vi "INST_PS_MEAS_3.0.0.vi"(0 "VISA session":refnum<visa-resource-name>="TCPIP0::169.254.70.130::inst0::INSTR", 1 "Clear Error in":bool, 3 "SEL_PS":string(combo)="PS1", 7 "Channel Name (1)":string="3", 11 "error in (no error)":errorcluster, 12 "Measurement Type (1: Voltage)":i32(ring)=1 items=["Current", "Voltage"], 14 "Use OPC?(T)":bool=TRUE) -> (4 "dup VISA session":refnum<visa-resource-name>="TCPIP0::169.254.70.130::inst0::INSTR", 6 "Measurement":dbl=28.01386 format="%.2p", 10 "Measurement (str)":string="+2.801386E+01\n", 15 "error out":errorcluster)   [LabVIEW 2018]
doc: "This VI takes a measurement on the output signal and returns the measured value."
uses:
  Initialize References/Station References Global.vi
panel:
  in  "General Settings:Timeout Value":u32=2000
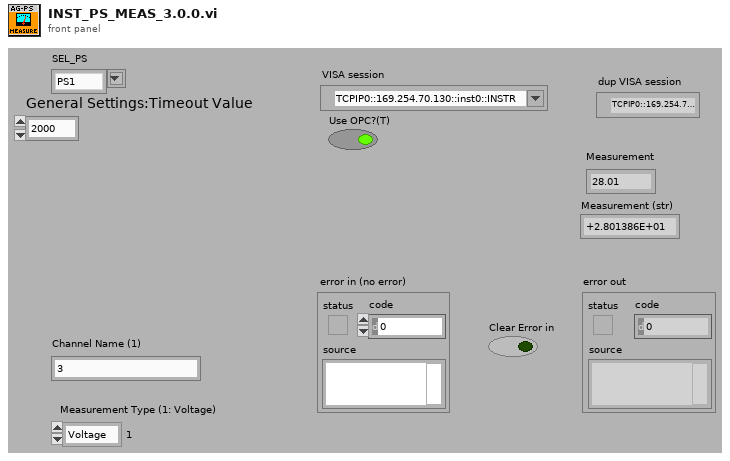
[diagram p1: front panel]
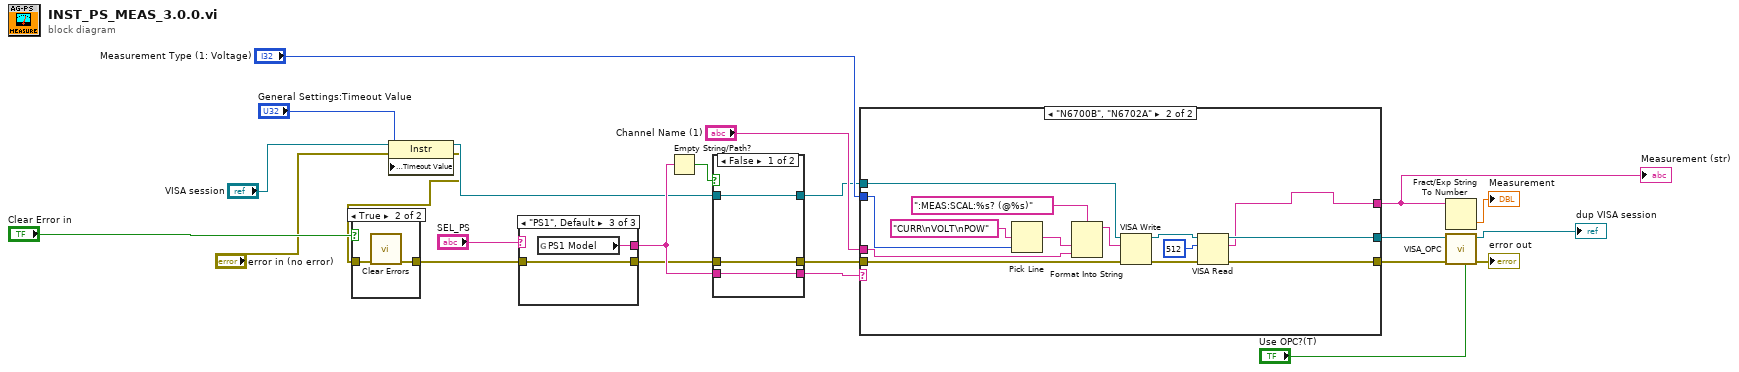
[diagram p0: block diagram]
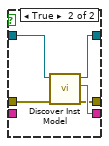
[diagram p2: hidden frame]
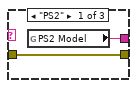
[diagram p3: hidden frame]
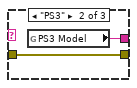
[diagram p4: hidden frame]
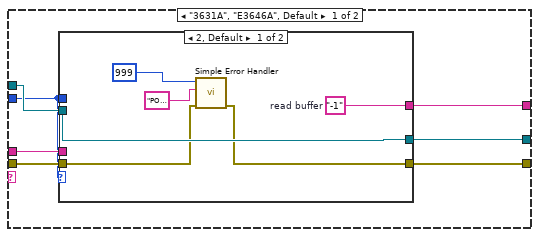
[diagram p5: hidden frame]
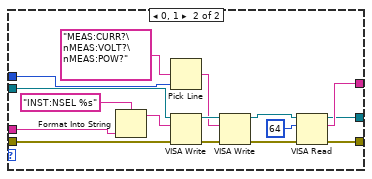
[diagram p6: hidden frame]
diagram:
  n1 = property class="Instr"(reference="VISA session", error in="error in (no error)", "General Settings:Timeout Value"="General Settings:Timeout Value") -> (reference out=w4:refnum<visa-resource-name>, error out=w3:errorcluster)
  n2 = case shown="True" "Clear Error in" {
    tunnel: w3 -> [w24 w26]
    tunnel: [w24 w25] -> w11
    frame False {
    }
    frame True {
      n3 = call <vilib>:"Clear Errors.vi"("error in (no error)"=w26) -> ("error out"=w25:errorcluster)  [unwired: 5 in, 1 out]
    }
  }
  n4 = case shown="\"PS1\", Default" "SEL_PS" {
    tunnel: [w28 w30 w32] -> w14
    tunnel: w11 -> [w27 w29 w31]
    tunnel: [w27 w29 w31] -> w13
    frame "PS2" {
      n5 = global read "Station References Global.vi" "PS2 Model"() -> (w28:string)
    }
    frame "PS3" {
      n6 = global read "Station References Global.vi" "PS3 Model"() -> (w30:string)
    }
    frame "PS1", Default {
      n7 = global read "Station References Global.vi" "PS1 Model"() -> (w32:string)
    }
  }
  n8 = Empty String/Path?(string/path=w14) -> (empty?=w15:bool)
  n9 = case shown="False" w15 {
    tunnel: [w35 w40] -> w9
    tunnel: w14 -> [w35 _]
    tunnel: [w34 w39] -> w10
    tunnel: w13 -> [w34 w38]
    tunnel: w4 -> [w33 w37]
    tunnel: [w33 w36] -> w8
    frame False {
    }
    frame True {
      n10 = call "Discover Inst Model.vi"("error in"=w38, "Session In"=w37) -> ("error out"=w39:errorcluster, "Model #"=w40:string, "Session Out"=w36:refnum<visa-resource-name>)  [unwired: 7 in]
    }
  }
  n11 = case shown="\"N6700B\", \"N6702A\"" w9 {
    tunnel: [w47 w71] -> w1
    tunnel: w8 -> [w46 w76]
    tunnel: [w45 w70] -> w23
    tunnel: [w44 w73] -> w20
    tunnel: w10 -> [w43 w72]
    tunnel: "Measurement Type (1: Voltage)" -> [w41 w75]
    tunnel: "Channel Name (1)" -> [w42 w74]
    frame "3631A", "E3646A", Default {
      n12 = case shown="2, Default" w41 {
        tunnel: [w52 w67] -> w47
        tunnel: w46 -> [w53 w61]
        tunnel: [w50 w60] -> w45
        tunnel: [w53 w59] -> w44
        tunnel: w43 -> [w51 w58]
        tunnel: w42 -> [_ w57]
        tunnel: w41 -> [_ w54]
        frame 2, Default {
          w52 = "-1"  # read buffer
          n13 = call <vilib>:"Simple Error Handler.vi"("error code (no error:0)"=999, "error source (\" \")"="POWER MEAS NOT AVAILABLE ON THIS MODEL OF PS" ("error source (\" \")"), "error in (no error)"=w51) -> ("error out"=w50:errorcluster)  [unwired: 2 in, 4 out]
        }
        frame 0, 1 {
          n14 = Format Into String(format string="INST:NSEL %s", w57) -> (resulting string=w64:string)  [unwired: 2 in, 1 out]
          n15 = Pick Line(multi-line string="MEAS:CURR?\nMEAS:VOLT?\nMEAS:POW?", line index=w54) -> (output string=w55:string)  [unwired: 1 in]
          n16 = VISA Write(VISA resource name=w61, write buffer=w64, error in (no error)=w58) -> (VISA resource name out=w62:refnum<visa-resource-name>, error out=w63:errorcluster)  [unwired: 1 out]
          n17 = VISA Write(VISA resource name=w62, write buffer=w55, error in (no error)=w63) -> (VISA resource name out=w66:refnum<visa-resource-name>, error out=w69:errorcluster)  [unwired: 1 out]
          n18 = VISA Read(VISA resource name=w66, byte count=u32 64, error in (no error)=w69) -> (VISA resource name out=w59:refnum<visa-resource-name>, read buffer=w67:string, error out=w60:errorcluster)  [unwired: 1 out]
        }
      }
    }
    frame "N6700B", "N6702A" {
      n19 = Pick Line(multi-line string="CURR\nVOLT\nPOW", line index=w75) -> (output string=w83:string)  [unwired: 1 in]
      n20 = Format Into String(format string=":MEAS:SCAL:%s? (@%s)", w83, w74) -> (resulting string=w82:string)  [unwired: 2 in, 1 out]
      n21 = VISA Write(VISA resource name=w76, write buffer=w82, error in (no error)=w72) -> (VISA resource name out=w80:refnum<visa-resource-name>, error out=w81:errorcluster)  [unwired: 1 out]
      n22 = VISA Read(VISA resource name=w80, byte count=u32 512, error in (no error)=w81) -> (VISA resource name out=w73:refnum<visa-resource-name>, read buffer=w71:string, error out=w70:errorcluster)  [unwired: 1 out]
    }
  }
  "Measurement (str)" <- w1
  n23 = Fract/Exp String To Number(string=w1) -> (number=→"Measurement":dbl)  [unwired: 3 in, 1 out]
  n24 = call "VISA_OPC.vi"("OPC(T)"="Use OPC?(T)", "error in"=w23, "Session In"=w20) -> ("error out"=→"error out":errorcluster, "Session Out"=→"dup VISA session":refnum<visa-resource-name>)  [unwired: 6 in, 1 out]
